vi "2-8.vi"() -> ()   [LabVIEW 2022 SP3]
uses:
  1e75b0b0-556f-43a4-9949-bbdf4f756169.vi
  <vilib>/Comparison/Less/Less Functor/Less Functor.lvclass
panel:
  out "最小值":dbl
  out "最大值":dbl
  out "从小到大排列":dbl[](array[numeric])
  out "倒序序列":dbl[](array[numeric])
  out "数组":dbl[](array[numeric])
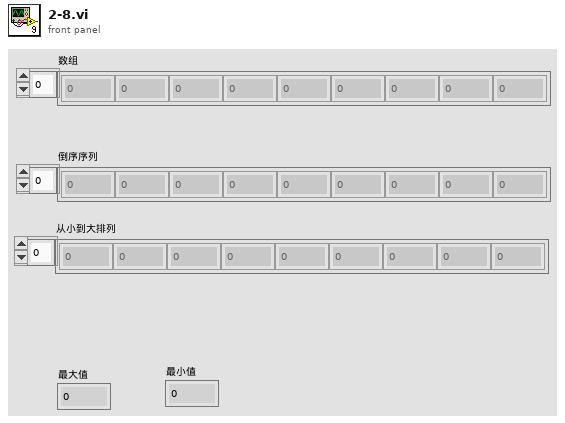
[diagram p1: front panel]
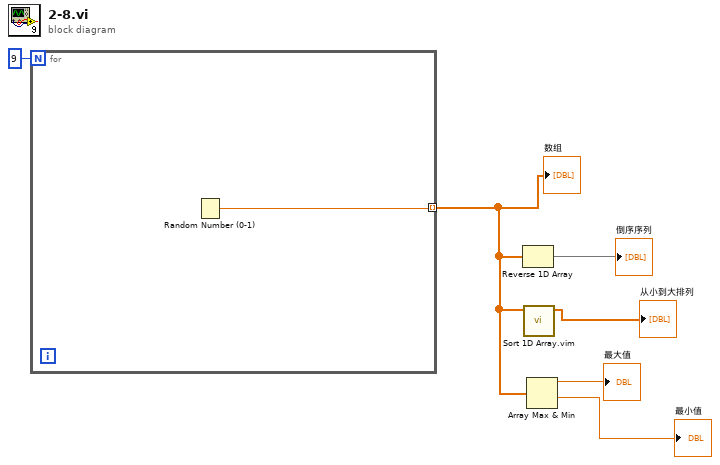
[diagram p0: block diagram]
diagram:
  n1 = for {
    N: 9 -> [_]
    tunnel: [w7] -> w3 mode=indexing
    n2 = Random Number (0-1)() -> (number: 0 to 1=w7:dbl)
  }
  "数组" <- w3
  n3 = Reverse 1D Array(array=w3) -> (reversed array=→"倒序序列":dbl[])
  n4 = call "Sort 1D Array.vim"("unsorted array"=w3) -> ("sorted array"=→"从小到大排列":dbl[])  [unwired: 10 in]
  n5 = Array Max & Min(array=w3) -> (max value=→"最大值":dbl, min value=→"最小值":dbl)  [unwired: 2 out]
